vi "Parse GPS_RAW_INT.vi"(11 "Data":string) -> (3 "GPS Data Out":T1)   [LabVIEW 2014]
uses:
  Aircraft Information/Controls/Aircraft GPS Data.ctl
panel:
  out "Satellites Visible":u8
  out "Fix Type":u8
  out "Course Over Ground (degrees)":u16
  out "GPS Ground Speed (m/s)":u16
  out "GPS VDOP (cm)":u16
  out "GPS HDOP (cm)":u16
  out "Altitude (m)":i32
  out "Longitude":i32
  out "Latitude (degrees)":i32
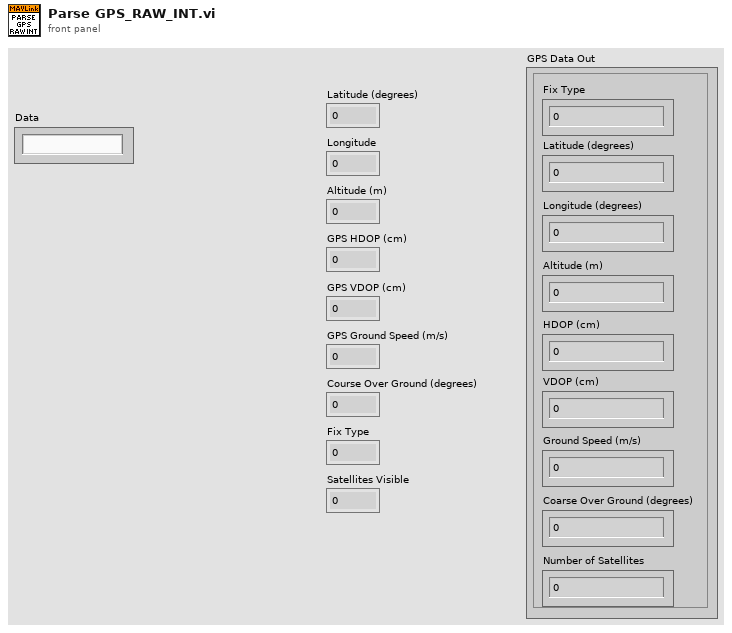
[diagram p1: front panel]
types:
  T1 = typedef "Aircraft GPS Data.ctl" = cluster{"Latitude (degrees)":dbl, "Longitude (degrees)":dbl, "Altitude (m)":dbl, "Fix Type":u8, "HDOP (cm)":u16, "VDOP (cm)":u16, "Ground Speed (m/s)":dbl, "Coarse Over Ground (degrees)":u16, "Number of Satellites":u8}
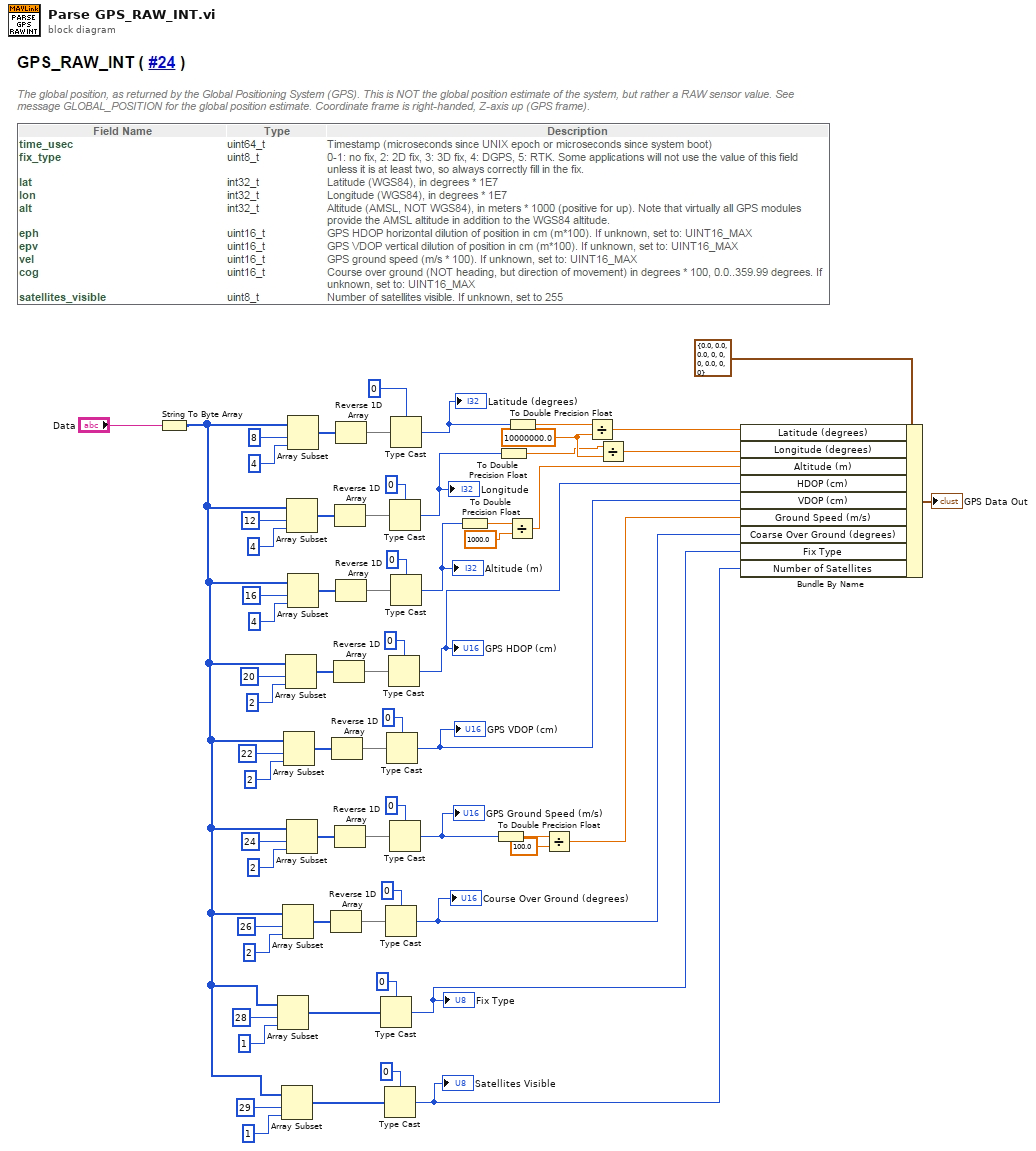
[diagram p0: block diagram]
diagram:
  w11 = 10000000.0 ("y")
  n1 = String To Byte Array(string="Data") -> (unsigned byte array=w23:u8[])
  n2 = Array Subset(array=w23, index=28, length=1) -> (w28:u8[])
  n3 = Array Subset(array=w23, index=29, length=1) -> (w27:u8[])
  n4 = Array Subset(array=w23, index=26, length=2) -> (w34:u8[])
  n5 = Array Subset(array=w23, index=22, length=2) -> (w44:u8[])
  n6 = Array Subset(array=w23, index=20, length=2) -> (w49:u8[])
  n7 = Array Subset(array=w23, index=12, length=4) -> (w58:u8[])
  n8 = Array Subset(array=w23, index=24, length=2) -> (w39:u8[])
  n9 = Array Subset(array=w23, index=8, length=4) -> (w65:u8[])
  n10 = Array Subset(array=w23, index=16, length=4) -> (w55:u8[])
  n11 = Reverse 1D Array(array=w34) -> (reversed array=w35:u8[])
  n12 = Reverse 1D Array(array=w44) -> (reversed array=w45:u8[])
  n13 = Reverse 1D Array(array=w49) -> (reversed array=w48:u8[])
  n14 = Reverse 1D Array(array=w58) -> (reversed array=w57:u8[])
  n15 = Reverse 1D Array(array=w39) -> (reversed array=w38:u8[])
  n16 = Reverse 1D Array(array=w65) -> (reversed array=w66:u8[])
  n17 = Reverse 1D Array(array=w55) -> (reversed array=w56:u8[])
  n18 = Type Cast(type=u8 0 ("single precision float"), x=w28) -> (*(type *) &x=w18:u8)
  "Fix Type" <- w18
  n19 = Type Cast(type=u8 0 ("single precision float"), x=w27) -> (*(type *) &x=w17:u8)
  "Satellites Visible" <- w17
  n20 = Type Cast(type=u16 0 ("single precision float"), x=w35) -> (*(type *) &x=w19:u16)
  "Course Over Ground (degrees)" <- w19
  n21 = Type Cast(type=u16 0 ("single precision float"), x=w45) -> (*(type *) &x=w20:u16)
  "GPS VDOP (cm)" <- w20
  n22 = Type Cast(type=u16 0 ("single precision float"), x=w48) -> (*(type *) &x=w21:u16)
  "GPS HDOP (cm)" <- w21
  n23 = Type Cast(type=0 ("single precision float"), x=w57) -> (*(type *) &x=w12:i32)
  "Longitude" <- w12
  n24 = Type Cast(type=u16 0 ("single precision float"), x=w38) -> (*(type *) &x=w8:u16)
  "GPS Ground Speed (m/s)" <- w8
  n25 = Type Cast(type=0 ("single precision float"), x=w66) -> (*(type *) &x=w15:i32)
  "Latitude (degrees)" <- w15
  n26 = Type Cast(type=0 ("single precision float"), x=w56) -> (*(type *) &x=w3:i32)
  "Altitude (m)" <- w3
  n27 = To Double Precision Float(number=w3) -> (double precision float=w4:dbl)
  n28 = To Double Precision Float(number=w8) -> (double precision float=w7:dbl)
  n29 = To Double Precision Float(number=w12) -> (double precision float=w10:dbl)
  n30 = Divide(x=w4, y=1000.0) -> (x/y=w1:dbl)
  n31 = To Double Precision Float(number=w15) -> (double precision float=w14:dbl)
  n32 = Divide(x=w7, y=100.0) -> (x/y=w5:dbl)
  n33 = Divide(x=w14, y=w11) -> (x/y=w13:dbl)
  n34 = Divide(x=w10, y=w11) -> (x/y=w9:dbl)
  n35 = Bundle By Name(cluster=T1 {"Latitude (degrees)"=0.0, "Longitude (degrees)"=0.0, "Altitude (m)"=0.0, "Fix Type"=0, "HDOP (cm)"=0, "VDOP (cm)"=0, "Ground Speed (m/s)"=0.0, "Coarse Over Ground (degrees)"=0, "Number of Satellites"=0} ("Aircraft GPS Data"), "Latitude (degrees)"=w13, "Longitude (degrees)"=w9, "Altitude (m)"=w1, "HDOP (cm)"=w21, "VDOP (cm)"=w20, "Ground Speed (m/s)"=w5, "Coarse Over Ground (degrees)"=w19, "Fix Type"=w18, "Number of Satellites"=w17) -> (→"GPS Data Out":T1)
